vi "Get Data Log Configuratuion.vi"(8 "error in (no error)":errorcluster) -> (0 "error out":errorcluster, 2 "Log Active":bool[][](array[boolean]), 3 "Log Headers":string[](array[string]))   [LabVIEW 2018]
uses:
  <vilib>/Utility/xml.llb/Read From XML File(string).vi
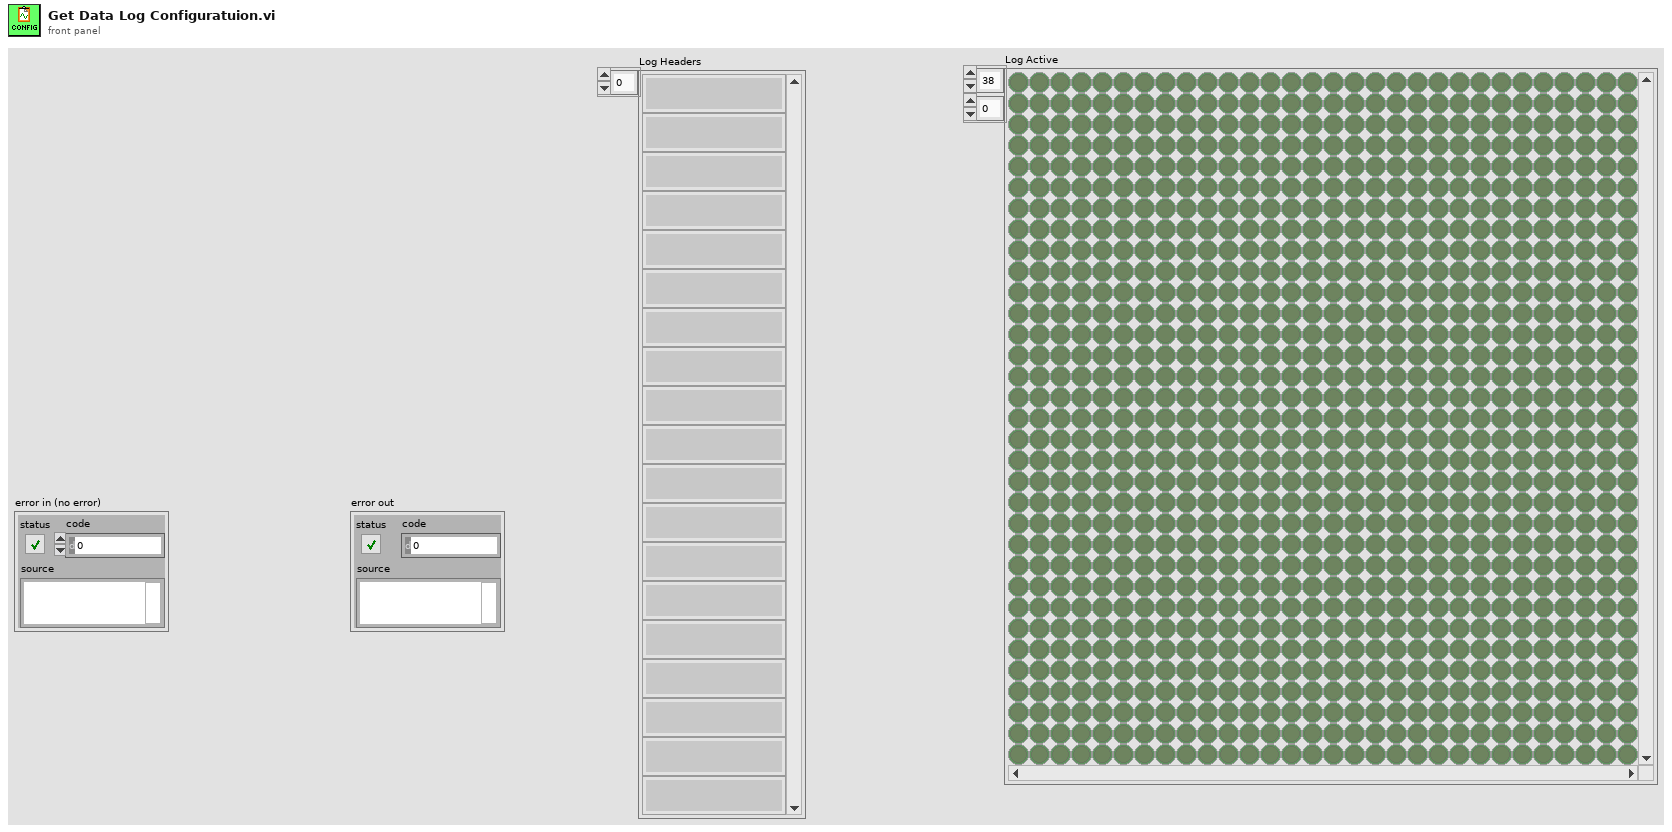
[diagram p1: front panel]
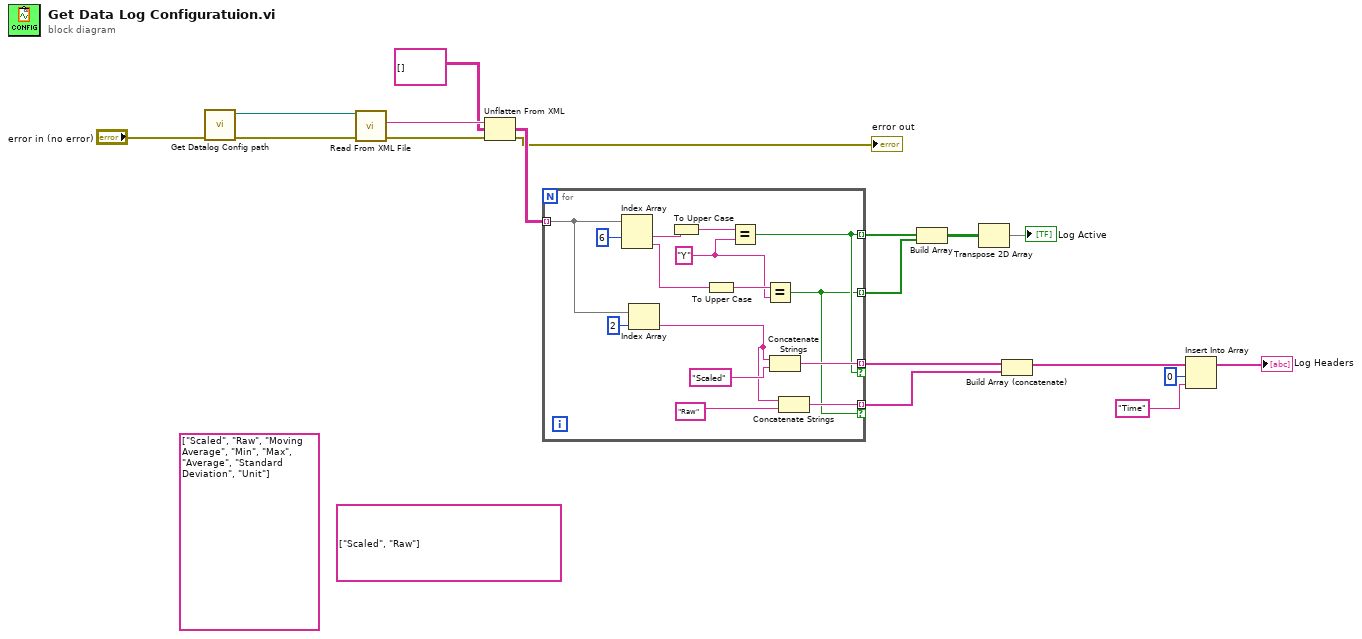
[diagram p0: block diagram]
diagram:
  (unwired) string[] ["Scaled", "Raw", "Moving Average", "Min", "Max", "Average", "Standard Deviation", "Unit"] ("Array")
  (unwired) string[] ["Scaled", "Raw"] ("Array")
  n1 = call "Get Datalog Config path.vi"("error in (no error)"="error in (no error)") -> ("error out"=w12:errorcluster, "Data Log Config"=w13:path)  [unwired: 9 in]
  n2 = call-poly <vilib>:"Read From XML File.vi"("error in (no error)"=w12, "XML File Path"=w13) -> ("error out"=w17:errorcluster, "XML Elements"=w18:string)  [unwired: 7 in, 1 out]
  n3 = Unflatten From XML(xml string=w18, type=string[][] [], error in (no error)=w17) -> (value=w15:string[][], error out=→"error out":errorcluster)
  n4 = for {
    tunnel: w15 -> [w30] mode=indexing
    tunnel: [w23] -> w4 mode=indexing
    tunnel: [w19] -> w3 mode=indexing
    tunnel: [w24] -> w7 mode=indexing if=w23
    tunnel: [w20] -> w6 mode=indexing if=w19
    w26 = "Y"
    n5 = Index Array(array=w30, index #1=6 ("disabled index (col)")) -> (element #1=w32:string, element #2=w27:string)  [unwired: 1 in]
    n6 = Index Array(array=w30, index=2) -> (element=w22:string)
    n7 = To Upper Case(1:w32) -> (0:w31:string)
    n8 = To Upper Case(1:w27) -> (0:w28:string)
    n9 = Equal?(x=w31, y=w26) -> (x = y?=w23:bool)
    n10 = Equal?(x=w28, y=w26) -> (x = y?=w19:bool)
    n11 = Concatenate Strings(w22, "Scaled") -> (w24:string)
    n12 = Concatenate Strings(w22, "Raw" ("String")) -> (w20:string)
  }
  n13 = Build Array(w4, w3) -> (w2:bool[][])
  n14 = Transpose 2D Array(2D array=w2) -> (transposed array=→"Log Active":bool[][])
  n15 = Build Array (concatenate)(w7, w6) -> (w5:string[])
  n16 = Insert Into Array(array=w5, index=0, new element="Time" ("new element/subarray")) -> (→"Log Headers":string[])
